vi "End Game.vi"(8 "error in (no error)":errorcluster, 11 "Map in":refnum<class "Map.lvclass">) -> (0 "error out":errorcluster, 3 "Map out":refnum<class "Map.lvclass">)   [LabVIEW 2020, in "SquareBattle.lvlib" / "Map.lvclass"]
uses:
  Map.lvclass
  Map.lvclass/Map.ctl
  Square/Square.lvclass
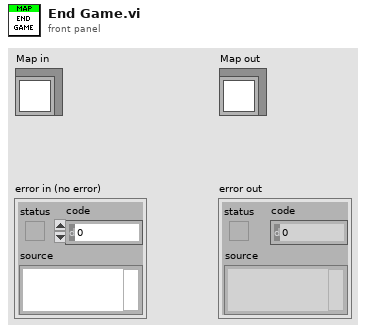
[diagram p1: front panel]
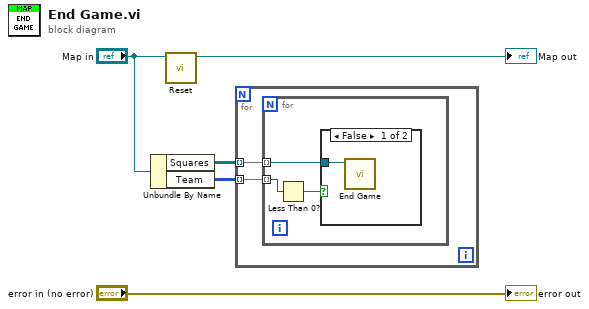
[diagram p0: block diagram]
diagram:
  n1 = Unbundle By Name("Map in") -> ("Squares"=w5:refnum<class "Square.lvclass">[][], "Team"=w4:i32[][])
  n2 = call "Reset.vi"("Map in"="Map in") -> ("Map out"=→"Map out":refnum<class "Map.lvclass">)  [unwired: 9 in, 1 out]
  n3 = for {
    tunnel: w5 -> [w7] mode=indexing
    tunnel: w4 -> [w6] mode=indexing
    n4 = for {
      tunnel: w7 -> [w8] mode=indexing
      tunnel: w6 -> [w10] mode=indexing
      n5 = Less Than 0?(x=w10) -> (x < 0?=w9:bool)
      n6 = case shown="False" w9 {
        tunnel: w8 -> [w11 _]
        frame False {
          n7 = call "End Game.vi"("Square in"=w11) -> ()  [unwired: 11 in]
        }
        frame True {
        }
      }
    }
  }
  "error out" <- "error in (no error)"
